vi "Explore Vertex.vi"(8 "Vertex":cluster{"row":i32, "col":i32}, 9 "Parent":cluster{"row":i32, "col":i32}, 10 "Map in":T1(c390), 11 "Queue in":refnum<queue>) -> (2 "Map out":T1(c390), 3 "Queue out":refnum<queue>)   [LabVIEW 2021, in "d12.lvlib"]
uses:
  d12.lvlib
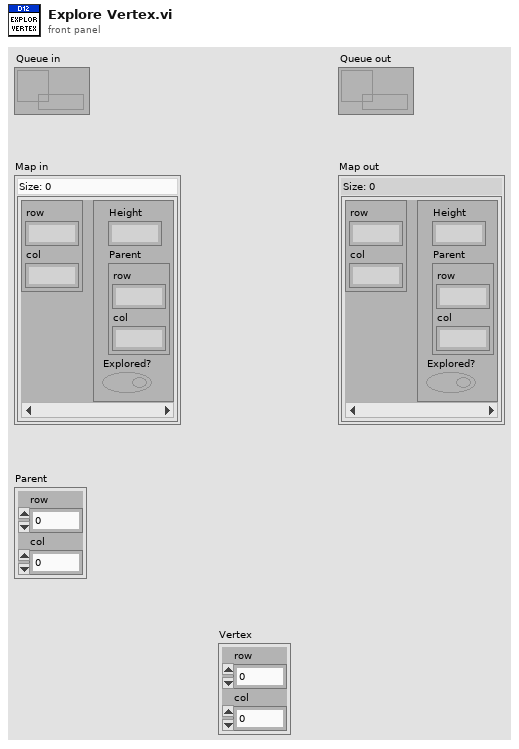
[diagram p1: front panel]
types:
  T1 = map{cluster{"row":i32, "col":i32}, cluster{"Height":i16, "Parent":cluster{"row":i32, "col":i32}, "Explored?":bool}}
  T2 = cluster{"Height":i16, "Parent":cluster{"row":i32, "col":i32}, "Explored?":bool}
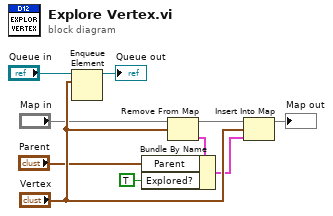
[diagram p0: block diagram]
diagram:
  n1 = Enqueue Element(queue="Queue in", element="Vertex") -> (queue out=→"Queue out":refnum<queue>)  [unwired: 2 in, 2 out]
  n2 = Remove From Map(10:"Vertex", 11:"Map in") -> (1:w6:T2, 3:w5:T1)  [unwired: 1 out]
  n3 = Bundle By Name(cluster=w6, "Parent"="Parent", "Explored?"=TRUE) -> (w7:T2)
  n4 = Insert Into Map(map in=w5, key="Vertex", value=w7) -> (map out=→"Map out":T1)  [unwired: 2 out]
